vi "Palettes to JSON.vi"(11 "Palettes":refnum<class "Material-Palette.lvclass">[](array[class])) -> (0 "error out":errorcluster, 3 "Material JSON":string)   [LabVIEW 2021, in "TSC Material Theme.lvlib" / "Material-Palette.lvclass"]
uses:
  Material-Palette.lvclass
  Material-Palette.lvclass/Material-Palette.ctl
  d83a044a-b5b8-4b98-af8e-c439c2b23e04.vi
  <vilib>/JDP Science/JSONtext/JSONtext.lvlib
  Serializer-Palette/Serializer-Palette.lvclass
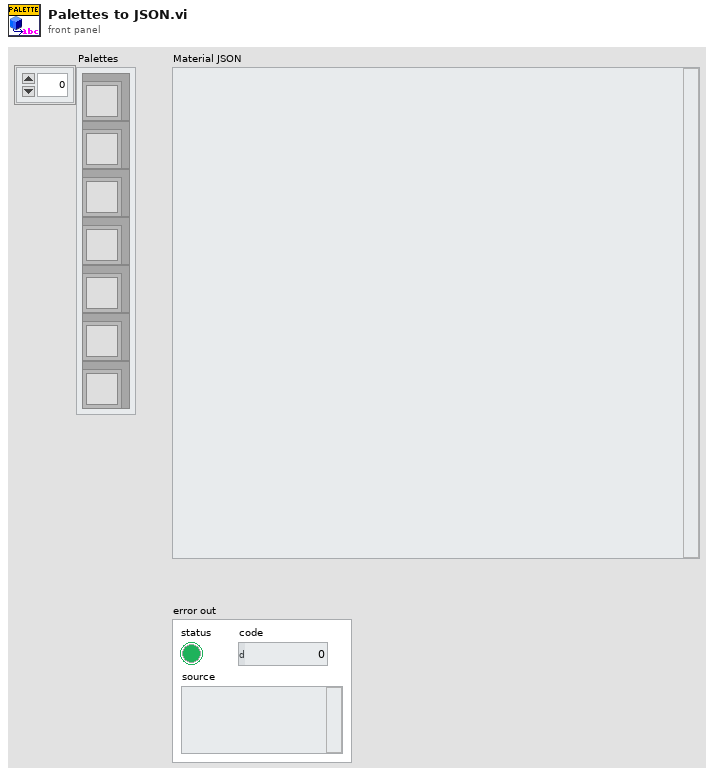
[diagram p1: front panel]
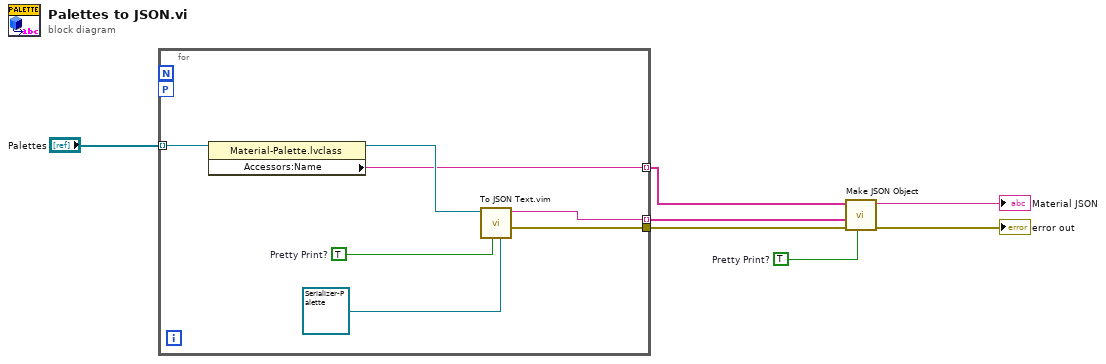
[diagram p0: block diagram]
diagram:
  w1 = TRUE  # Pretty Print?
  n1 = for {
    tunnel: [w14] -> w7
    workers-P: _ -> [_]
    tunnel: "Palettes" -> [w12] mode=indexing
    tunnel: [w10] -> w4 mode=indexing
    tunnel: [w9] -> w3 mode=indexing
    w8 = TRUE  # Pretty Print?
    n2 = property class="Material-Palette.lvclass"(reference=w12) -> (reference out=w11:refnum<class "Material-Palette.lvclass">, "Accessors:Name"=w9:string)  [unwired: 1 in, 1 out]
    n3 = call "To JSON Text.vim"("LVClass Serializer"=refnum<class "Serializer-Palette.lvclass"> refnum ("TSC Material Theme.lvlib:Class 1.lvclass"), "Pretty Print?"=w8, "Anything"=w11) -> ("error out"=w14:errorcluster, "<JSON>"=w10:string)  [unwired: 7 in]
  }
  n4 = call <vilib>:"Make JSON Object.vi"("Pretty Print?"=w1, "error in (no error)"=w7, "JSON Items"=w4, "Item Names"=w3) -> ("error out"=→"error out":errorcluster, "<JSON>"=→"Material JSON":string)  [unwired: 6 in]
